vi "USRP_freqsweepUSRP1.vi"() -> ()   [LabVIEW 2021]
uses:
  <vilib>/addons/Modulation/Analog/controls/Complex Data Waveform.ctl
  <vilib>/measure/maspectr.llb/Power Spectrum and PSD Export Mode.ctl
  system stop.vi
  <vilib>/measure/matone.llb/Extract Single Tone Information 1 Chan (CDB).vi
  <vilib>/measure/maspectr.llb/FFT Power Spectrum and PSD for 1 Chan (CDB).vi
  <instrlib>/niUSRP/niUSRP Fetch Rx Data (CDB Cluster).vi
  <instrlib>/niUSRP/niUSRP Write Tx Data (CDB Cluster).vi
  <vilib>/addons/Modulation/niAMT.lvlib
  <vilib>/measure/NI_MAPro.lvlib
panel:
  in  "Tab Control":T1(tab)
  in  "IQ rate Tx":dbl=100000.0 format="%#_6p"
  in  "Tx Gain":dbl format="%#_6f"
  in  "Tx IP":refnum<k15>
  out "coerced IQ rate Tx":dbl=100000.0 format="%#_6p"
  out "coerced carrier frequency Tx":dbl=100000.0 format="%#_6p"
  in  "Rx IP":refnum<k15>
  in  "Rx gain":dbl format="%#_6f"
  in  "Frequency":dbl format="%#_13g"
  in  "Duration":dbl format="%#_13g"
  out "coerced IQ rate Rx":dbl=100000.0 format="%#_6p"
  out "coerced carrier frequency Rx":dbl=100000.0 format="%#_6p"
  in  "number of samples":i64=100000
  out "Waveform Graph":dbl[](graph)
  out "Boolean":bool
  out "Received Waveform Graph":cluster{"f0":dbl, "df":dbl, "magnitude":dbl[]}(graph)
  out "detected frequency":dbl format="%.2p"
  out "detected Amplitude in dBm":dbl format="%.2p"
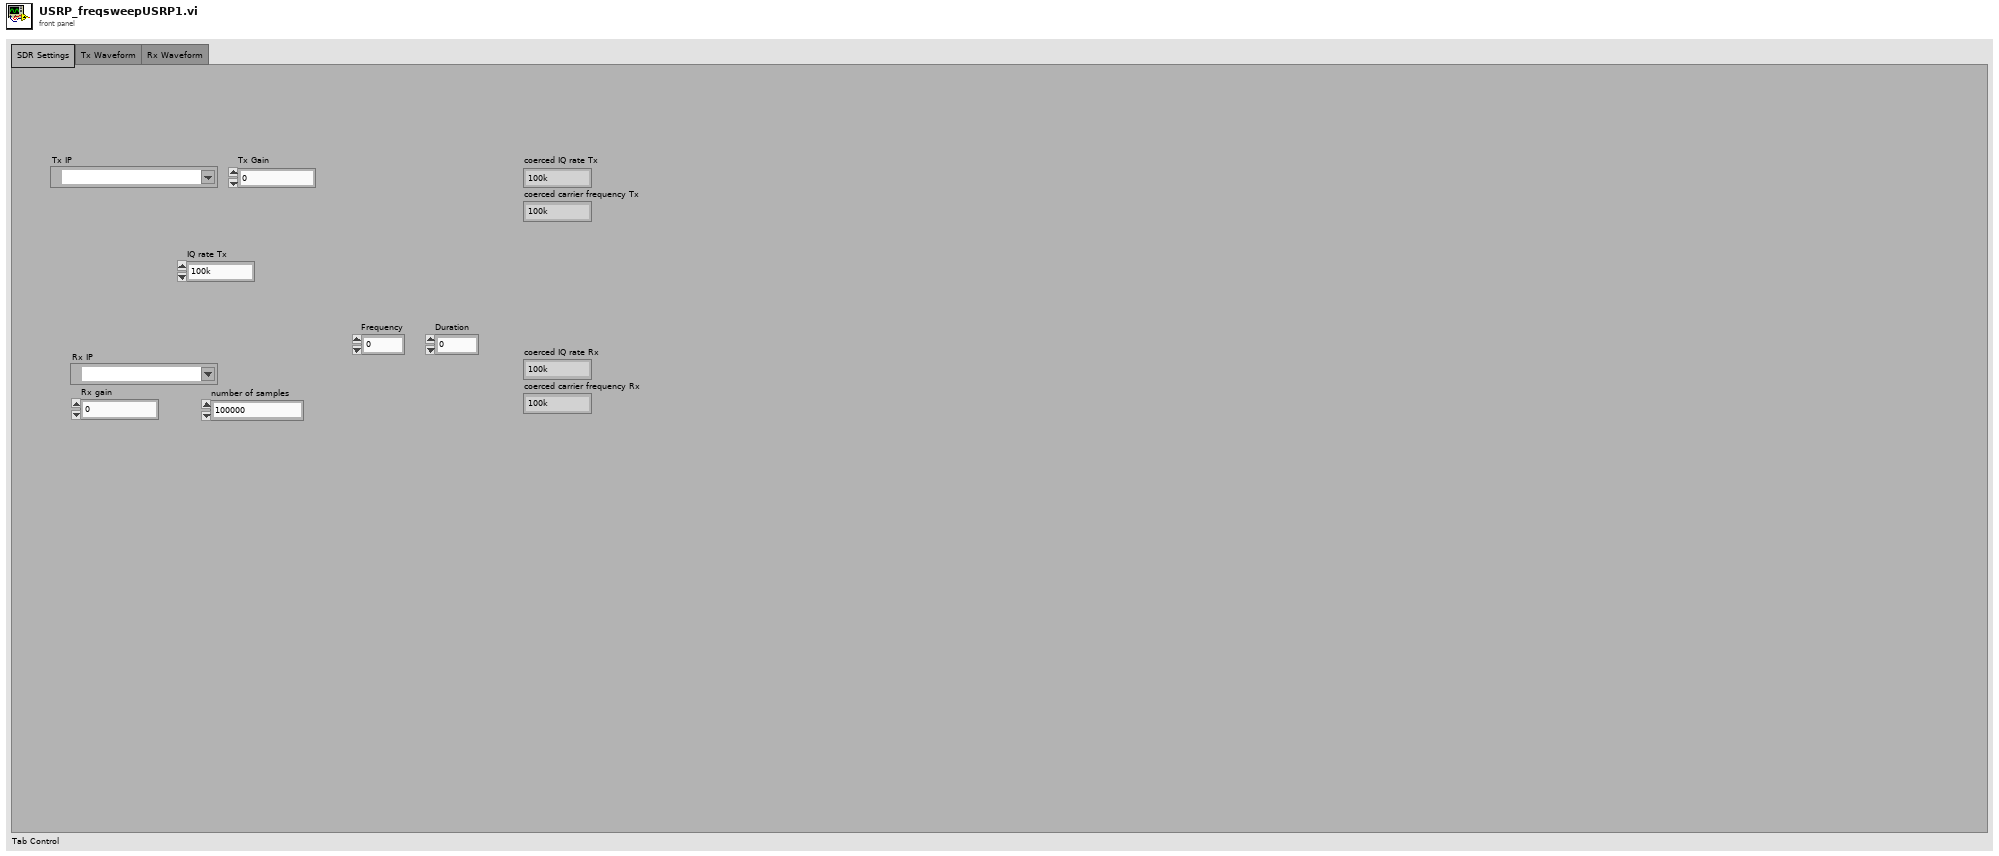
[diagram p1: front panel]
types:
  T1 = enum32{"SDR Settings", "Tx Waveform", "Rx Waveform"}
  T2 = typedef "niAMT.lvlib/Complex Data Waveform.ctl" = cluster{"t0":dbl, "dt":dbl, "Y":cdb[]}
  T3 = typedef "NI_MAPro.lvlib/Power Spectrum and PSD Export Mode.ctl" = u16
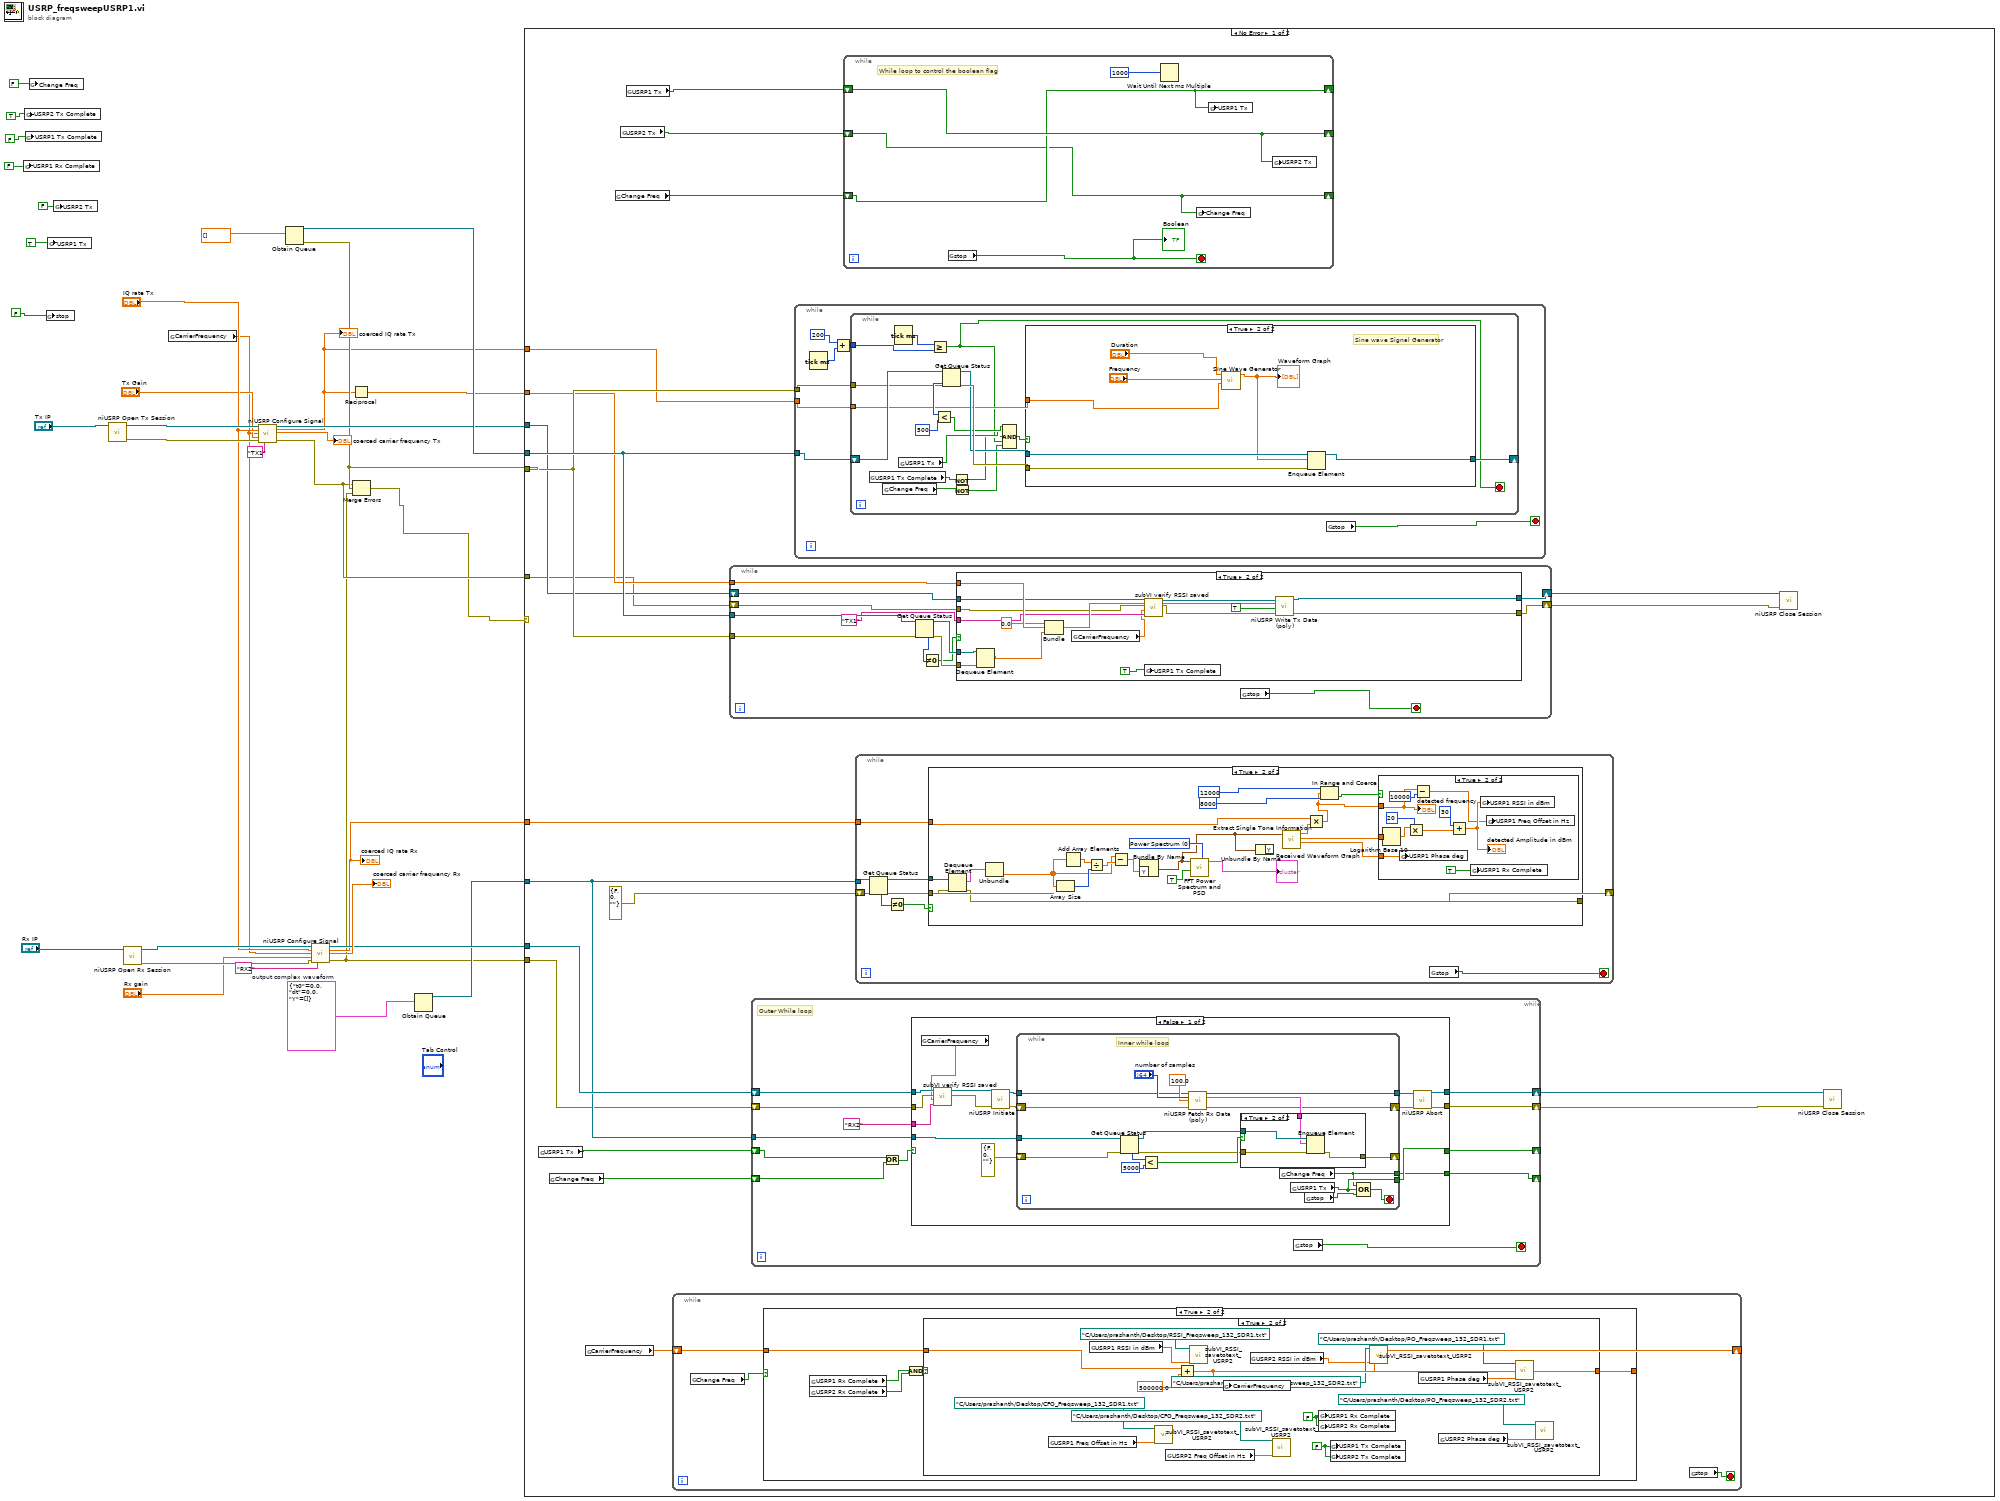
[diagram p0: block diagram]
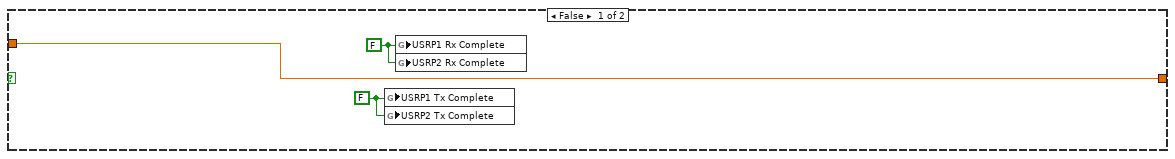
[diagram p3: hidden frame]
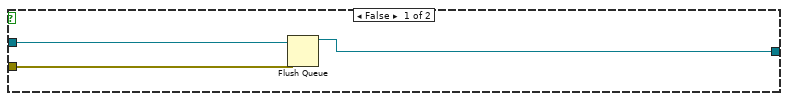
[diagram p4: hidden frame]
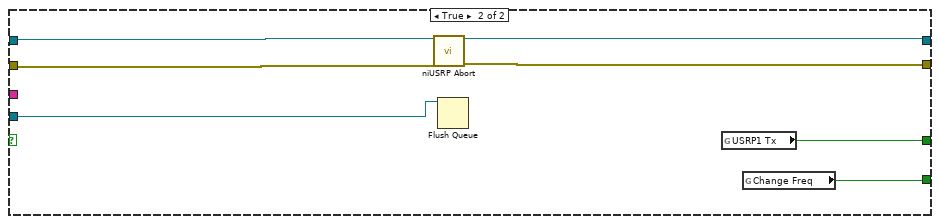
[diagram p6: hidden frame]
diagram:
  w8 = T2 {"t0"=0.0, "dt"=0.0, "Y"=[]}  # output complex waveform
  n1 = global write "system stop.vi" "USRP1 Rx Complete"(FALSE) -> ()
  n2 = global write "system stop.vi" "USRP2 Tx Complete"(TRUE) -> ()
  n3 = global write "system stop.vi" "USRP1 Tx Complete"(FALSE) -> ()
  n4 = global write "system stop.vi" "Change Freq"(FALSE) -> ()
  n5 = global write "system stop.vi" "stop"(FALSE) -> ()
  n6 = global write "system stop.vi" "USRP1 Tx"(TRUE) -> ()
  n7 = global write "system stop.vi" "USRP2 Tx"(FALSE) -> ()
  n8 = call <instrlib>:"niUSRP Open Tx Session.vi"("device names"="Tx IP") -> ("session handle out"=w33:refnum<k15>, "error out"=w32:errorcluster)  [unwired: 13 in]
  n9 = call <instrlib>:"niUSRP Open Rx Session.vi"("device names"="Rx IP") -> ("session handle out"=w30:refnum<k15>, "error out"=w29:errorcluster)  [unwired: 13 in]
  n10 = global read "system stop.vi" "CarrierFrequency"() -> (w3:dbl)
  n11 = call <instrlib>:"niUSRP Configure Signal.vi"("session handle"=w33, "IQ rate"="IQ rate Tx", "carrier frequency"=w3, "gain"="Tx Gain", "error in (no error)"=w32, "active antenna"="TX1") -> ("session handle out"=w15:refnum<k15>, "coerced IQ rate"=w12:dbl, "coerced carrier frequency"=→"coerced carrier frequency Tx":dbl, "error out"=w11:errorcluster)  [unwired: 5 in, 1 out]
  "coerced IQ rate Tx" <- w12
  n12 = Obtain Queue(element data type=dbl[] []) -> (queue out=w16:refnum<queue>, error out=w13:errorcluster)  [unwired: 4 in, 1 out]
  n13 = call <instrlib>:"niUSRP Configure Signal.vi"("session handle"=w30, "IQ rate"="IQ rate Tx", "carrier frequency"=w3, "gain"="Rx gain", "error in (no error)"=w29, "active antenna"="RX2") -> ("session handle out"=w9:refnum<k15>, "coerced IQ rate"=w6:dbl, "coerced carrier frequency"=→"coerced carrier frequency Rx":dbl, "error out"=w4:errorcluster)  [unwired: 5 in, 1 out]
  "coerced IQ rate Rx" <- w6
  n14 = Reciprocal(x=w12) -> (1/x=w14:dbl)
  n15 = Merge Errors(w11, w13, w4) -> (w2:errorcluster)
  n16 = Obtain Queue(element data type=w8) -> (queue out=w7:refnum<queue>)  [unwired: 4 in, 2 out]
  n17 = case shown="No Error" w2 {
    tunnel: w13 -> [w54 _]
    tunnel: w16 -> [w55 _]
    tunnel: w15 -> [w52 _]
    tunnel: w14 -> [w53 _]
    tunnel: w12 -> [w51 _]
    tunnel: w11 -> [w50 _]
    tunnel: w9 -> [w48 _]
    tunnel: w7 -> [w47 _]
    tunnel: w6 -> [w46 _]
    tunnel: w4 -> [w45 _]
    frame No Error {
      n18 = global read "system stop.vi" "USRP1 Tx"() -> (w44:bool)
      n19 = global read "system stop.vi" "Change Freq"() -> (w35:bool)
      n20 = global read "system stop.vi" "CarrierFrequency"() -> (w36:dbl)
      n21 = global read "system stop.vi" "Change Freq"() -> (w37:bool)
      n22 = global read "system stop.vi" "USRP2 Tx"() -> (w42:bool)
      n23 = global read "system stop.vi" "USRP1 Tx"() -> (w43:bool)
      n24 = while {
        shift-right: [w57] -> _
        shift-left: w36 -> [w58]
        stop <- w56 stop-if-true
        n25 = global read "system stop.vi" "Change Freq"() -> (w59:bool)
        n26 = case shown="True" w59 {
          tunnel: w58 -> [w60 w62]
          tunnel: [w60 w61] -> w57
          frame False {
          }
          frame True {
            n27 = global read "system stop.vi" "USRP1 Rx Complete"() -> (w65:bool)
            n28 = global read "system stop.vi" "USRP2 Rx Complete"() -> (w64:bool)
            n29 = And(x=w65, y=w64) -> (x .and. y?=w63:bool)
            n30 = case shown="True" w63 {
              tunnel: w62 -> [w68 w84]
              tunnel: [w68 w81] -> w61
              frame False {
                w67 = FALSE
                w66 = FALSE
                n31 = global write "system stop.vi" "USRP1 Tx Complete"(w67) -> ()
                n32 = global write "system stop.vi" "USRP2 Tx Complete"(w67) -> ()
                n33 = global write "system stop.vi" "USRP1 Rx Complete"(w66) -> ()
                n34 = global write "system stop.vi" "USRP2 Rx Complete"(w66) -> ()
              }
              frame True {
                w83 = FALSE
                w82 = FALSE
                n35 = global read "system stop.vi" "USRP1 Freq Offset in Hz"() -> (w75:dbl)
                n36 = global read "system stop.vi" "USRP1 RSSI in dBm"() -> (w79:dbl)
                n37 = call "subVI_RSSI_savetotext_USRP2.vi"("RSSI"=w75, "file path (dialog if empty)"=path "C:/Users/prashanth/Desktop/CFO_Freqsweep_132_SDR1.txt") -> ()  [unwired: 10 in]
                n38 = global read "system stop.vi" "USRP2 Freq Offset in Hz"() -> (w73:dbl)
                n39 = Add(x=w84, y=500000.0) -> (x+y=w81:dbl)
                n40 = call "subVI_RSSI_savetotext_USRP2.vi"("RSSI"=w79, "file path (dialog if empty)"=path "C:/Users/prashanth/Desktop/RSSI_Freqsweep_132_SDR1.txt") -> ()  [unwired: 10 in]
                n41 = global write "system stop.vi" "CarrierFrequency"(w81) -> ()
                n42 = global read "system stop.vi" "USRP2 RSSI in dBm"() -> (w77:dbl)
                n43 = call "subVI_RSSI_savetotext_USRP2.vi"("RSSI"=w73, "file path (dialog if empty)"=path "C:/Users/prashanth/Desktop/CFO_Freqsweep_132_SDR2.txt") -> ()  [unwired: 10 in]
                n44 = global write "system stop.vi" "USRP1 Rx Complete"(w82) -> ()
                n45 = global write "system stop.vi" "USRP2 Rx Complete"(w82) -> ()
                n46 = global write "system stop.vi" "USRP1 Tx Complete"(w83) -> ()
                n47 = global write "system stop.vi" "USRP2 Tx Complete"(w83) -> ()
                n48 = call "subVI_RSSI_savetotext_USRP2.vi"("RSSI"=w77, "file path (dialog if empty)"=path "C:/Users/prashanth/Desktop/RSSI_Freqsweep_132_SDR2.txt") -> ()  [unwired: 10 in]
                n49 = global read "system stop.vi" "USRP1 Phase deg"() -> (w71:dbl)
                n50 = global read "system stop.vi" "USRP2 Phase deg"() -> (w69:dbl)
                n51 = call "subVI_RSSI_savetotext_USRP2.vi"("RSSI"=w71, "file path (dialog if empty)"=path "C:/Users/prashanth/Desktop/PO_Freqsweep_132_SDR1.txt") -> ()  [unwired: 10 in]
                n52 = call "subVI_RSSI_savetotext_USRP2.vi"("RSSI"=w69, "file path (dialog if empty)"=path "C:/Users/prashanth/Desktop/PO_Freqsweep_132_SDR2.txt") -> ()  [unwired: 10 in]
              }
            }
          }
        }
        n53 = global read "system stop.vi" "stop"() -> (w56:bool)
      }
      n54 = while {
        tunnel: w55 -> [w239]
        tunnel: w54 -> [w236]
        tunnel: w53 -> [w235]
        shift-right: [w232] -> w39
        shift-left: w52 -> [w228]
        shift-right: [w231] -> w38
        shift-left: w50 -> [w227]
        stop <- w230 stop-if-true
        n55 = Get Queue Status(queue=w239, error in (no error)=w236) -> (queue out=w238:refnum<queue>, error out=w237:errorcluster, # elements in queue=w234:i32)  [unwired: 1 in, 5 out]
        n56 = Not Equal To 0?(x=w234) -> (x != 0?=w233:bool)
        n57 = case shown="True" w233 {
          tunnel: w238 -> [_ w257]
          tunnel: w237 -> [_ w256]
          tunnel: w235 -> [_ w255]
          tunnel: w228 -> [w241 w244]
          tunnel: w227 -> [w240 w243]
          tunnel: [w241 w251] -> w232
          tunnel: [w240 w249] -> w231
          tunnel: "TX1" ("Configuration:Active Antenna") -> [_ w247]
          frame False {
          }
          frame True {
            n58 = Dequeue Element(queue=w257, error in (no error)=w256) -> (element=w248:dbl[])  [unwired: 1 in, 3 out]
            n59 = Bundle(0.0, w255, w248) -> (w254:cluster{dbl, dbl, dbl[]})  [unwired: 1 in]
            n60 = global read "system stop.vi" "CarrierFrequency"() -> (w242:dbl)
            n61 = call "subVI verify RSSI saved.vi"("Configuration:Active Antenna"=w247, "Configuration:Carrier Frequency"=w242, "error in (no error)"=w243, "reference"=w244) -> ("error out"=w246:errorcluster, "reference out"=w245:refnum<k15>)  [unwired: 6 in]
            n62 = global write "system stop.vi" "USRP1 Tx Complete"(TRUE) -> ()
            n63 = call-poly <instrlib>:"niUSRP Write Tx Data (poly).vi"("session handle"=w245, "data"=w254, "end of data?"=TRUE, "error in (no error)"=w246) -> ("session handle out"=w251:refnum<k15>, "error out"=w249:errorcluster)  [unwired: 10 in]
          }
        }
        n64 = global read "system stop.vi" "stop"() -> (w230:bool)
      }
      n65 = while {
        tunnel: w47 -> [w137]
        shift-right: [w134] -> _
        shift-left: w44 -> [w132]
        shift-right: [w136] -> w41
        shift-left: w48 -> [w127]
        shift-right: [w135] -> w40
        shift-left: w45 -> [w126]
        shift-right: [w130] -> _
        shift-left: w35 -> [w129]
        stop <- w133 stop-if-true
        # "Outer While loop"
        n66 = Or(x=w132, y=w129) -> (x .or. y?=w131:bool)
        n67 = case shown="False" w131 {
          tunnel: w127 -> [w140 w183]
          tunnel: w137 -> [w153 w179]
          tunnel: w126 -> [w139 w181]
          tunnel: [w147 w182] -> w136
          tunnel: [w146 w180] -> w135
          tunnel: [w151 w184] -> w134
          tunnel: [w144 w178] -> w130
          tunnel: "RX2" ("Configuration:Active Antenna") -> [w143 _]
          frame False {
            n68 = global read "system stop.vi" "CarrierFrequency"() -> (w138:dbl)
            n69 = call "subVI verify RSSI saved.vi"("Configuration:Active Antenna"=w143, "Configuration:Carrier Frequency"=w138, "error in (no error)"=w139, "reference"=w140) -> ("error out"=w142:errorcluster, "reference out"=w141:refnum<k15>)  [unwired: 6 in]
            n70 = call <instrlib>:"niUSRP Initiate.vi"("session handle"=w141, "error in (no error)"=w142) -> ("session handle out"=w150:refnum<k15>, "error out"=w149:errorcluster)  [unwired: 12 in]
            n71 = while {
              tunnel: w153 -> [w172]
              shift-right: [w156] -> w145
              shift-left: w149 -> [w158]
              shift-right: [w171] -> _
              shift-left: errorcluster {"status"=FALSE, "code"=0, "source"=""} ("error in (no error)") -> [w170]
              tunnel: [w155] -> w151
              tunnel: w150 -> [w159]
              tunnel: [w157] -> w148
              tunnel: [w154] -> w144
              stop <- w162 stop-if-true
              # "Inner while loop"
              n72 = Get Queue Status(queue=w172, error in (no error)=w170) -> (queue out=w165:refnum<queue>, error out=w166:errorcluster, # elements in queue=w169:i32)  [unwired: 1 in, 5 out]
              n73 = Less?(x=w169, y=5000) -> (x < y?=w167:bool)
              n74 = call-poly <instrlib>:"niUSRP Fetch Rx Data (poly).vi"("session handle"=w159, "number of samples"="number of samples", "timeout"=100.0, "error in (no error)"=w158) -> ("session handle out"=w157:refnum<k15>, "data"=w163:cluster{"t0":dbl, "dt":dbl, "Y":cdb[]}, "error out"=w156:errorcluster)  [unwired: 8 in, 1 out]
              n75 = case shown="True" w167 {
                tunnel: w166 -> [w173 w177]
                tunnel: w165 -> [_ w176]
                tunnel: w163 -> [_ w175]
                tunnel: [w173 w174] -> w171
                frame False {
                }
                frame True {
                  n76 = Enqueue Element(queue=w176, element=w175, error in (no error)=w177) -> (error out=w174:errorcluster)  [unwired: 1 in, 2 out]
                }
              }
              n77 = global read "system stop.vi" "Change Freq"() -> (w154:bool)
              n78 = global read "system stop.vi" "USRP1 Tx"() -> (w155:bool)
              n79 = global read "system stop.vi" "stop"() -> (w161:bool)
              n80 = Compound Arithmetic op=OR(w154, w155, w161) -> (w162:bool)
            }
            n81 = call <instrlib>:"niUSRP Abort.vi"("session handle"=w148, "error in (no error)"=w145) -> ("session handle out"=w147:refnum<k15>, "error out"=w146:errorcluster)  [unwired: 12 in]
          }
          frame True {
            n82 = call <instrlib>:"niUSRP Abort.vi"("session handle"=w183, "error in (no error)"=w181) -> ("session handle out"=w182:refnum<k15>, "error out"=w180:errorcluster)  [unwired: 12 in]
            n83 = Flush Queue(queue=w179) -> ()  [unwired: 1 in, 3 out]
            n84 = global read "system stop.vi" "USRP1 Tx"() -> (w184:bool)
            n85 = global read "system stop.vi" "Change Freq"() -> (w178:bool)
          }
        }
        n86 = global read "system stop.vi" "stop"() -> (w133:bool)
      }
      n87 = while {
        tunnel: w55 -> [w97]
        tunnel: w54 -> [w96]
        tunnel: w51 -> [w95]
        stop <- w91 stop-if-true
        n88 = Tick Count (ms)() -> (millisecond timer value=w93:u32)
        n89 = Add(x=200, y=w93) -> (x+y=w92:u32)
        n90 = while {
          tunnel: w96 -> [w110]
          tunnel: w95 -> [w109]
          tunnel: w92 -> [w104]
          shift-right: [w102] -> _
          shift-left: w97 -> [w111]
          stop <- w99 stop-if-true
          n91 = global read "system stop.vi" "USRP1 Tx Complete"() -> (w101:bool)
          n92 = global read "system stop.vi" "Change Freq"() -> (w100:bool)
          n93 = Tick Count (ms)() -> (millisecond timer value=w105:u32)
          n94 = global read "system stop.vi" "USRP1 Tx"() -> (w107:bool)
          n95 = Greater Or Equal?(x=w105, y=w104) -> (x >= y?=w99:bool)
          n96 = Get Queue Status(queue=w111, error in (no error)=w110) -> (queue out=w112:refnum<queue>, error out=w113:errorcluster, # elements in queue=w115:i32)  [unwired: 1 in, 5 out]
          n97 = Less?(x=w115, y=500) -> (x < y?=w108:bool)
          n98 = Not(x=w101) -> (.not. x?=w103:bool)
          n99 = Not(x=w100) -> (.not. x?=w98:bool)
          n100 = Compound Arithmetic op=AND(w108, w107, w103, w99, w98) -> (w106:bool)
          n101 = case shown="True" w106 {
            tunnel: w113 -> [w117 w125]
            tunnel: w112 -> [w118 w124]
            tunnel: w109 -> [_ w121]
            tunnel: [w116 w120] -> w102
            frame False {
              n102 = Flush Queue(queue=w118, error in (no error)=w117) -> (queue out=w116:refnum<queue>)  [unwired: 2 out]
            }
            frame True {
              # "Sine wave Signal Generator"
              n103 = call "SIne Wave Generator.vi"("Sampling rate"=w121, "Frequency"="Frequency", "Duration"="Duration") -> ("Array"=w119:dbl[])  [unwired: 7 in, 1 out]
              "Waveform Graph" <- w119
              n104 = Enqueue Element(queue=w124, element=w119, error in (no error)=w125) -> (queue out=w120:refnum<queue>)  [unwired: 1 in, 2 out]
            }
          }
        }
        n105 = global read "system stop.vi" "stop"() -> (w91:bool)
      }
      n106 = while {
        shift-right: [w87] -> _
        shift-left: w43 -> [w89]
        shift-right: [w89] -> _
        shift-left: w42 -> [w86]
        shift-right: [w86] -> _
        shift-left: w37 -> [w87]
        stop <- w88 stop-if-true
        # "While loop to control the boolean flag"
        n107 = global read "system stop.vi" "stop"() -> (w88:bool)
        "Boolean" <- w88
        n108 = Wait Until Next ms Multiple(millisecond multiple=1000) -> ()  [unwired: 1 out]
        n109 = global write "system stop.vi" "Change Freq"(w86) -> ()
        n110 = global write "system stop.vi" "USRP1 Tx"(w87) -> ()
        n111 = global write "system stop.vi" "USRP2 Tx"(w89) -> ()
      }
      n112 = while {
        tunnel: w47 -> [w190]
        shift-right: [w187] -> _
        shift-left: errorcluster {"status"=FALSE, "code"=0, "source"=""} ("error in (no error)") -> [w189]
        tunnel: w46 -> [w186]
        stop <- w185 stop-if-true
        n113 = Get Queue Status(queue=w190, error in (no error)=w189) -> (queue out=w192:refnum<queue>, error out=w191:errorcluster, # elements in queue=w193:i32)  [unwired: 1 in, 5 out]
        n114 = Not Equal To 0?(x=w193) -> (x != 0?=w188:bool)
        n115 = case shown="True" w188 {
          tunnel: w192 -> [_ w215]
          tunnel: w191 -> [w194 w210]
          tunnel: [w194 w208] -> w187
          tunnel: w186 -> [_ w199]
          frame False {
          }
          frame True {
            w212 = T3 0 items=["Power Spectrum", "Power Spectral Density"] ("export mode")
            n116 = Dequeue Element(queue=w215, error in (no error)=w210) -> (element=w209:T2, error out=w208:errorcluster)  [unwired: 1 in, 2 out]
            n117 = Unbundle(w209) -> ("Y"=w204:cdb[])  [unwired: 2 out]
            n118 = Array Size(array=w204) -> (size(s)=w206:i32)
            n119 = Add Array Elements(numeric array=w204) -> (sum=w207:cdb)
            n120 = Divide(x=w207, y=w206) -> (x/y=w205:cdb)
            n121 = Subtract(x=w204, y=w205) -> (x-y=w203:cdb[])
            n122 = Bundle By Name("Y"=w203) -> (w211:waveform(cdb))  [unwired: 1 in]
            n123 = call-poly <vilib>:"FFT Power Spectrum and PSD.vi"("export mode"=w212, "dB On (F)"=TRUE, "time signal"=w211) -> ("Power Spectrum / PSD"=→"Received Waveform Graph":cluster{"f0":dbl, "df":dbl, "magnitude":dbl[]})  [unwired: 5 in, 3 out]
            n124 = Unbundle By Name(w211) -> ()  [unwired: 1 out]
            n125 = call-poly <vilib>:"Extract Single Tone Information.vi"("time signal in"=w211) -> ("detected phase (deg)"=w195:dbl, "detected amplitude"=w197:dbl, "detected frequency"=w200:dbl)  [unwired: 5 in, 3 out]
            n126 = Multiply(x=w199, y=w200) -> (x*y=w196:dbl)
            n127 = In Range and Coerce(upper limit=12000, x=w196, lower limit=8000) -> (In Range?=w198:bool)  [unwired: 1 out]
            n128 = case shown="True" w198 {
              tunnel: w197 -> [_ w224]
              tunnel: w196 -> [_ w219]
              tunnel: w195 -> [_ w216]
              frame False {
              }
              frame True {
                n129 = Logarithm Base 10(1:w224) -> (0:w226:dbl)
                n130 = global write "system stop.vi" "USRP1 Phase deg"(w216) -> ()
                n131 = Multiply(x=w226, y=20) -> (x*y=w222:dbl)
                n132 = Subtract(x=w219, y=10000) -> (x-y=w217:dbl)
                n133 = Add(x=30, y=w222) -> (x+y=w220:dbl)
                "detected Amplitude in dBm" <- w220
                n134 = global write "system stop.vi" "USRP1 Rx Complete"(TRUE) -> ()
                n135 = global write "system stop.vi" "USRP1 RSSI in dBm"(w220) -> ()
                n136 = global write "system stop.vi" "USRP1 Freq Offset in Hz"(w217) -> ()
                "detected frequency" <- w219
              }
            }
          }
        }
        n137 = global read "system stop.vi" "stop"() -> (w185:bool)
      }
      n138 = call <instrlib>:"niUSRP Close Session.vi"("session handle"=w39, "error in (no error)"=w38) -> ()  [unwired: 13 in, 1 out]
      n139 = call <instrlib>:"niUSRP Close Session.vi"("session handle"=w41, "error in (no error)"=w40) -> ()  [unwired: 13 in, 1 out]
    }
    frame Error {
    }
  }
